vi "New-Window.vi"(8 "error in (no error)":errorcluster, 10 "View":refnum<class "View.lvclass">) -> (0 "error out":errorcluster, 3 "Window":refnum<class "Window.lvclass">)   [LabVIEW 2024, in "GLF.lvlib" / "Window.lvclass"]
uses:
  Window.lvclass
  View/View.lvclass
  Window.lvclass/Window.ctl
  DVR--cluster.ctl
  <vilib>/Saukko/LV SDL3/Sources/SDL3/Video/WindowID--integer.ctl
  <vilib>/Saukko/LV SDL3/Sources/SDL3/Video/Video.lvlib
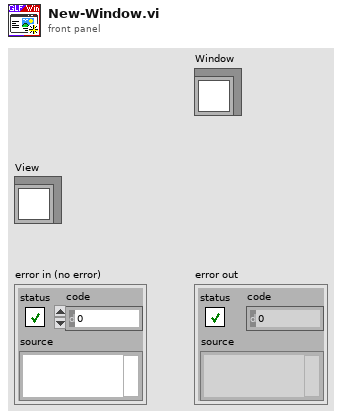
[diagram p1: front panel]
types:
  T1 = typedef "GLF.lvlib/Window.lvclass/DVR--cluster.ctl" = cluster{"SDL_Window *":i64, "Window ID":T2}
  T2 = typedef "SDL3.lvlib/Video.lvlib/WindowID--integer.ctl" = u32
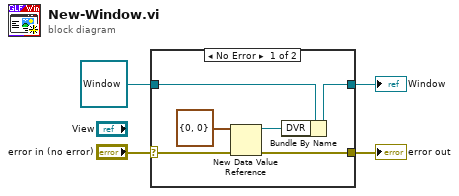
[diagram p0: block diagram]
diagram:
  n1 = case shown="No Error" "error in (no error)" {
    selector: "error in (no error)" -> [w8 w12]
    tunnel: [w5 w12] -> w3
    tunnel: [w7 w11] -> w1
    tunnel: refnum<class "Window.lvclass"> refnum ("Window in") -> [w6 w11]
    frame No Error {
      n2 = New Data Value Reference(data value=T1 {"SDL_Window *"=0, "Window ID"=0} ("DVR"), error in=w8) -> (data value reference=w10:refnum<data-value>, error out=w5:errorcluster)
      n3 = Bundle By Name(cluster=w6, "DVR"=w10) -> (w7:refnum<class "Window.lvclass">)
    }
    frame Error {
    }
  }
  "error out" <- w3
  "Window" <- w1
